vi "global.vi"() -> ()   [LabVIEW 2011]
panel:
  in  "Bandwidth":string(combo)="125"
  in  "CRC":bool
  in  "Preamble length":u32=8 max=65535 step=1
  in  "Frequency":u32=57600 max=65535 step=1
  in  "Bitrate":u32=50000 max=65535 step=1
  in  "Freq deviation":u32=57600 max=65535 step=1
  in  "RX signal bw":string(combo)
  in  "Freq correct":string(combo)
  in  "Spreading factor":string(combo)
  in  "Power":string(combo)
  in  "Radio mode":string(combo)
  out "Get RW param":bool
  out "Get RO param":bool
  # "Device history config"
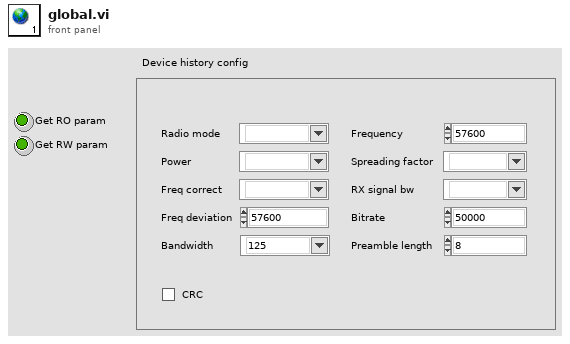
[diagram p1: front panel]
diagram:
